vi "output_tunnel.vi"() -> ()   [LabVIEW 2021]
panel:
  out "Conditional":i32[][](array[numeric])
  out "Concatenating":i32[](array[numeric])
  out "Indexing":i32[][](array[numeric])
  out "Last Value":i32[](array[numeric])
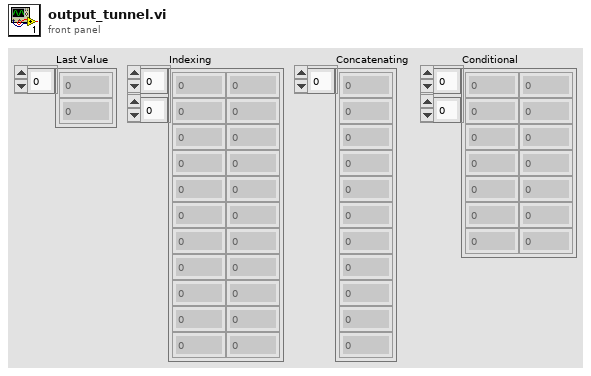
[diagram p1: front panel]
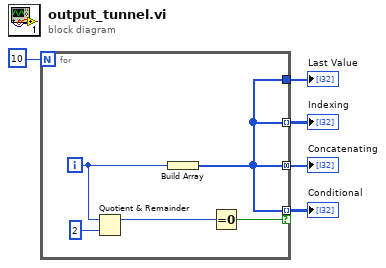
[diagram p0: block diagram]
diagram:
  n1 = for {
    N: 10 -> [_]
    tunnel: [w10] -> w4
    tunnel: [w10] -> w3 mode=indexing
    tunnel: [w10] -> w2 mode=concatenating
    tunnel: [w10] -> w1 mode=indexing if=w6
    i -> [w9]
    n2 = Quotient & Remainder(x=w9, y=2) -> (x-y*floor(x/y)=w7:i32)  [unwired: 1 out]
    n3 = Build Array "Build Array"(w9) -> (w10:i32[])
    n4 = Equal To 0?(x=w7) -> (x = 0?=w6:bool)
  }
  "Last Value" <- w4
  "Indexing" <- w3
  "Concatenating" <- w2
  "Conditional" <- w1
